vi "Write to Hardware.vi"(7 "valid triggers":bool, 8 "error in":errorcluster, 9 "trigger values":dbl[](array[numeric]), 10 "values in":dbl[](array[numeric]), 11 "execution unit in":refnum<class "Execution Unit.lvclass">) -> (0 "error out":errorcluster, 1 "trigger values out":dbl[](array[numeric]), 2 "values out":dbl[](array[numeric]), 3 "execution unit out":refnum<class "Execution Unit.lvclass">)   [LabVIEW 2020, in "Ballard ARINC 429 Engine.lvlib" / "Interfaces.lvlib" / "Execution Unit.lvclass"]
uses:
  Execution Unit.lvclass
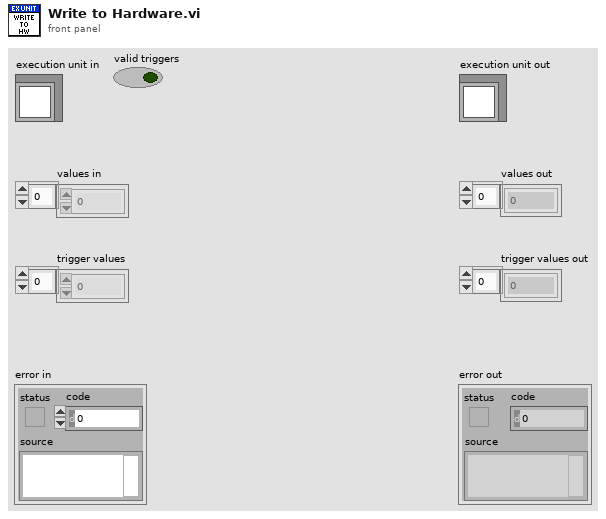
[diagram p1: front panel]
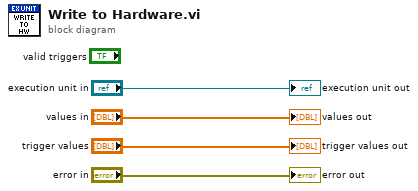
[diagram p0: block diagram]
diagram:
  "error out" <- "error in"
  "execution unit out" <- "execution unit in"
  "values out" <- "values in"
  "trigger values out" <- "trigger values"
